vi "Xbox Vibration.vi"(1 "Rough Vibration":u16, 2 "Smooth Vibration":u16, 3 "dwUserIndex":u32) -> ()   [LabVIEW 2015]
doc: "Makes the controller with the user index specified (0/1/2/3) vibrade (in two diffent vibration methodes).\n~~~~~~~~~~~~~~~~PAY ATTENTION! ~~~~~~~~~~~~~~~~\nRequires to install the XInput shared library (instructions in Google Drive > General Angels #2230 2014 > úåëðä > Programming Progress Logs > [E] Library > Controller > Xbox Vibration > Imprting XInput Shared Library."
uses:
  <userlib>/xinput1_3/xinput1_3.lvlib
panel:
  in  "pVibration":T1 {"wLeftMotorSpeed (Rough)" scale=0.0..65536.0; "wRightMotorSpeed  (Smooth)" scale=0.0..65536.0}
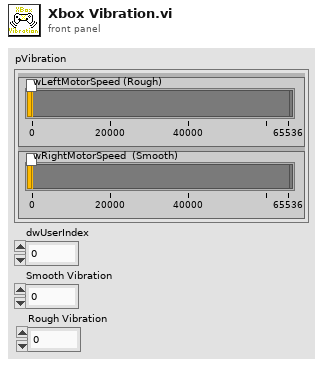
[diagram p1: front panel]
types:
  T1 = cluster{"wLeftMotorSpeed (Rough)":u16, "wRightMotorSpeed  (Smooth)":u16}
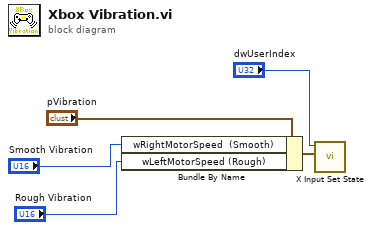
[diagram p0: block diagram]
diagram:
  n1 = Bundle By Name(cluster="pVibration", "wRightMotorSpeed  (Smooth)"="Smooth Vibration", "wLeftMotorSpeed (Rough)"="Rough Vibration") -> (w3:T1)
  n2 = call <userlib>:"X Input Set State.vi"("pVibration"=w3, "dwUserIndex"="dwUserIndex") -> ()  [unwired: 8 in, 2 out]
